vi "Measurement.GetPublicEventsRegistration.vi"(8 "error in (no error)":errorcluster, 11 "Measurement in":refnum<class "Measurement.lvclass">) -> (0 "error out":errorcluster, 2 "Measurement Public Events":refnum<event-registration>, 3 "Measurement out":refnum<class "Measurement.lvclass">)   [LabVIEW 2017, in "Measurement.lvclass"]
uses:
  Measurement.lvclass
  Typedefs/PublicEvents--Cluster.ctl
  Typedefs/PublicEvents--Measurement.Initialized.ctl
  Typedefs/Measurement.Measured--Data.ctl
  Typedefs/PublicEvents--Measurement.Uninitialized.ctl
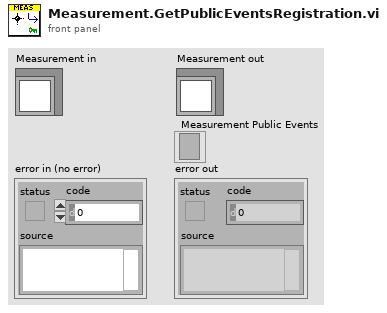
[diagram p1: front panel]
types:
  T1 = typedef "Measurement.lvclass/PublicEvents--Cluster.ctl" = cluster{"Initialized":refnum<user-event>, "Measured":refnum<user-event>, "Uninitialized":refnum<user-event>}
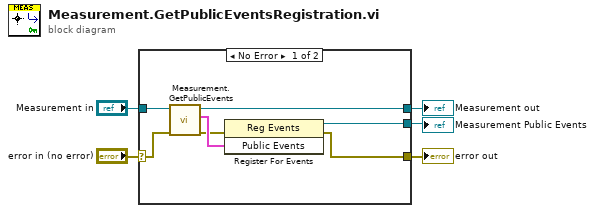
[diagram p0: block diagram]
diagram:
  n1 = case shown="No Error" "error in (no error)" {
    selector: "error in (no error)" -> [w11 w14]
    tunnel: [w7 w14] -> w4
    tunnel: [w6 w13] -> w2
    tunnel: "Measurement in" -> [w12 w13]
    tunnel: [w8 _] -> w1
    frame No Error {
      n2 = call "Measurement.GetPublicEvents.vi"("error in (no error)"=w11, "Measurement in"=w12) -> ("error out"=w9:errorcluster, "Public Events"=w10:T1, "Measurement out"=w6:refnum<class "Measurement.lvclass">)  [unwired: 7 in]
      n3 = register-events(error in=w9, w10) -> (reference out=w8:refnum<event-registration>, error out=w7:errorcluster)  [unwired: 1 in]
    }
    frame Error {
    }
  }
  "error out" <- w4
  "Measurement out" <- w2
  "Measurement Public Events" <- w1
